vi "LM get new coefficients.vi"(0 "Coefficients":dbl[](array[numeric]) format="%0.2f", 1 "lamda":dbl=100.0 format="%0.2e", 5 "Alpha":T1, 7 "Beta":dbl[](array[numeric]) format="%.6e", 11 "error in (no error)":errorcluster) -> (4 "New Coefficients":dbl[](array[numeric]) format="%0.2f", 15 "error out":errorcluster)   [LabVIEW 2010, in "NI_Gmath.lvlib"]
uses:
  NI_Gmath.lvlib
  RealMatrix.ctl
  Matrix left divisionMV.vi
  NI_Matrix.lvlib
panel:
  # "Get New Coefficients"
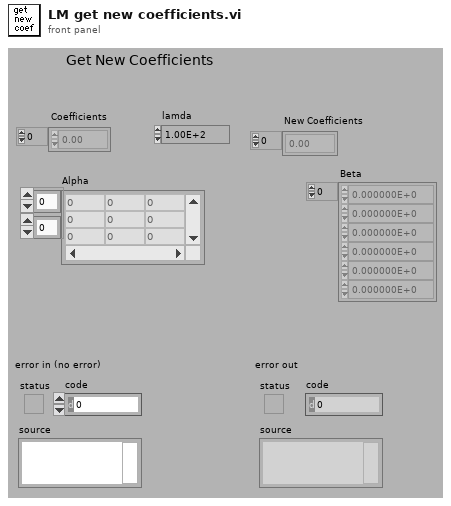
[diagram p1: front panel]
types:
  T1 = typedef "NI_Matrix.lvlib/RealMatrix.ctl" = dbl[][]
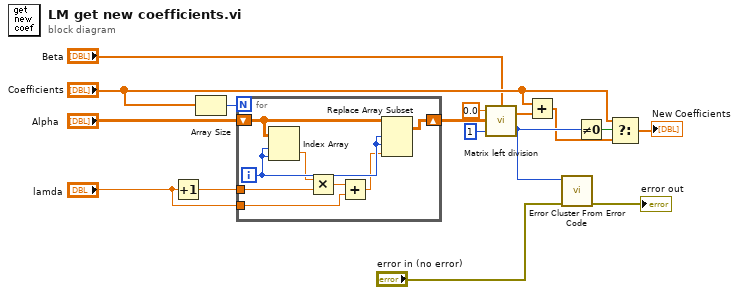
[diagram p0: block diagram]
diagram:
  n1 = Increment(x="lamda") -> (x+1=w7:dbl)
  n2 = Array Size(array="Coefficients") -> (size(s)=w15:i32)
  n3 = for {
    N: w15 -> [_]
    shift-right: [w20] -> w5
    shift-left: "Alpha" -> [w24]
    tunnel: w7 -> [w22]
    tunnel: "lamda" -> [w21]
    i -> [w23]
    n4 = Index Array(array=w24, index (row)=w23, index (col)=w23) -> (element=w18:dbl)
    n5 = Multiply(x=w18, y=w22) -> (x*y=w17:dbl)
    n6 = Add(x=w17, y=w21) -> (x+y=w19:dbl)
    n7 = Replace Array Subset(array=w24, new element=w19, index (row)=w23, index (col)=w23) -> (w20:T1)
  }
  n8 = call-poly "Matrix left division.vi"("A"="Beta", "number of iterations"=1, "B"=w5, "SVD relative tolerance"=0.0) -> ("error"=w16:i32, "B\\A"=w3:dbl[])
  n9 = Add(x="Coefficients", y=w3) -> (x+y=w14:dbl[])
  n10 = call "Error Cluster From Error Code.vi"("error in (no error)"="error in (no error)", "error code (0)"=w16) -> ("error out"=→"error out":errorcluster)  [unwired: 7 in]
  n11 = Not Equal To 0?(x=w16) -> (x != 0?=w9:bool)
  n12 = Select(t="Coefficients", s=w9, f=w14) -> (s? t:f=→"New Coefficients":dbl[])
